vi "Read Read after write.vi"(11 "Device in":refnum<class "Device.lvclass">) -> (2 "Read after write":bool=TRUE, 3 "Device out":refnum<class "Device.lvclass">)   [LabVIEW 2020, in "Device.lvclass"]
uses:
  Device.lvclass
  Device.lvclass/Device.ctl
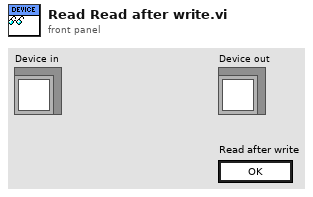
[diagram p1: front panel]
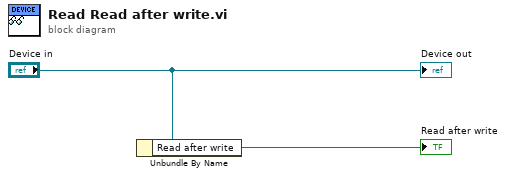
[diagram p0: block diagram]
diagram:
  n1 = Unbundle By Name("Device in") -> ("Read after write"=→"Read after write":bool)
  "Device out" <- "Device in"
